vi "ADD OF 2D NUMBER(SubVI).vi"(6 "B in":dbl, 7 "A in":dbl) -> (0 "B out":bool[][](array[boolean]), 1 "A+B 2":dbl, 2 "A+B":bool[][](array[boolean]), 3 "A out":bool[][](array[boolean]))   [LabVIEW 2019]
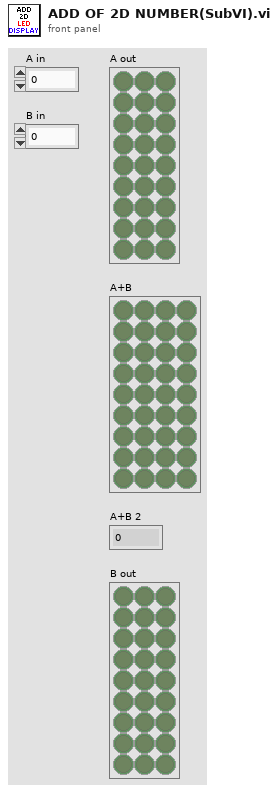
[diagram p1: front panel]
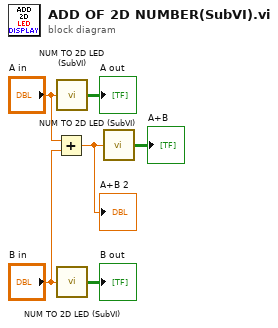
[diagram p0: block diagram]
diagram:
  n1 = Add(x="A in", y="B in") -> (x+y=w4:dbl)
  "A+B 2" <- w4
  n2 = call "NUM TO 2D LED (SubVI).vi"("A"="A in") -> ("transposed array"=→"A out":bool[][])
  n3 = call "NUM TO 2D LED (SubVI).vi"("A"="B in") -> ("transposed array"=→"B out":bool[][])
  n4 = call "NUM TO 2D LED (SubVI).vi"("A"=w4) -> ("transposed array"=→"A+B":bool[][])
